vi "My Nonlinear Curve Fit LM bounds.vi"(0 "Y":dbl[](array[numeric]), 1 "f(x,a)":T5, 2 "data":variant, 5 "X":dbl[](array[numeric]), 7 "Weight":dbl[](array[numeric]), 9 "initial parameters":dbl[](array[numeric]), 11 "error in (no error)":errorcluster, 12 "Termination Criteria":T6={"Max Iterations"=1000, "Max Function Calls"=10000, "Max Time"=1000.0, "Function Tolerance"=1e-06, "Parameter Tolerance"=1e-06, "Gradient Tolerance"=1e-06, "Min Lambda"=1e-06, "Max Lambda"=1000000.0, "Initial Tick Count"=0}, 13 "parameter bounds":T3, 14 "method":T4 items=["Least Square", "Least Absolute Residual", "Bisquare"]) -> (3 "Fit Aborted?":bool, 4 "best nonlinear fit":dbl[](array[numeric]), 6 "best fit parameters":dbl[](array[numeric]), 8 "covariance":T7, 10 "Fit Statistics":T1, 15 "error out":errorcluster)   [LabVIEW 2019]
uses:
  <vilib>/Analysis/Matrix/Datatypes/RealMatrix.ctl
  My Fit Stopping Criteria.ctl
  <vilib>/gmath/NumericalOptimization/LM model function reference.ctl
  <vilib>/Analysis/6fits.llb/Curve Fitting Criteria.ctl
  Fit Statistics.ctl
  Convergence Criteria.ctl
  <vilib>/gmath/NumericalOptimization/LM model function.ctl
  <vilib>/gmath/NumericalOptimization/LM_output select.ctl
  Abort Fit Global.vi
  <vilib>/gmath/NI_Gmath.lvlib
  <vilib>/Analysis/NI_AALBase.lvlib
  <vilib>/Analysis/Matrix/NI_Matrix.lvlib
  <vilib>/Analysis/NI_AALPro.lvlib
panel:
  out "Lambda Chart":dbl(graph)
  out "Parameters Gradient Chart":dbl[][](graph)
  in  "Repeat Fit N times (2)":i32=2
  in  "Reset Charts":bool
  out "Chi2 Chart":dbl(graph)
  out "Parameters Graph":dbl[](graph)
  in  "Delay (ms)":i32
  in  "Debug":bool
  out "Parameters Chart":dbl[][](graph)
  out "Function & Fit Graph":cluster{"New Coefficients":dbl[]}[](graph)
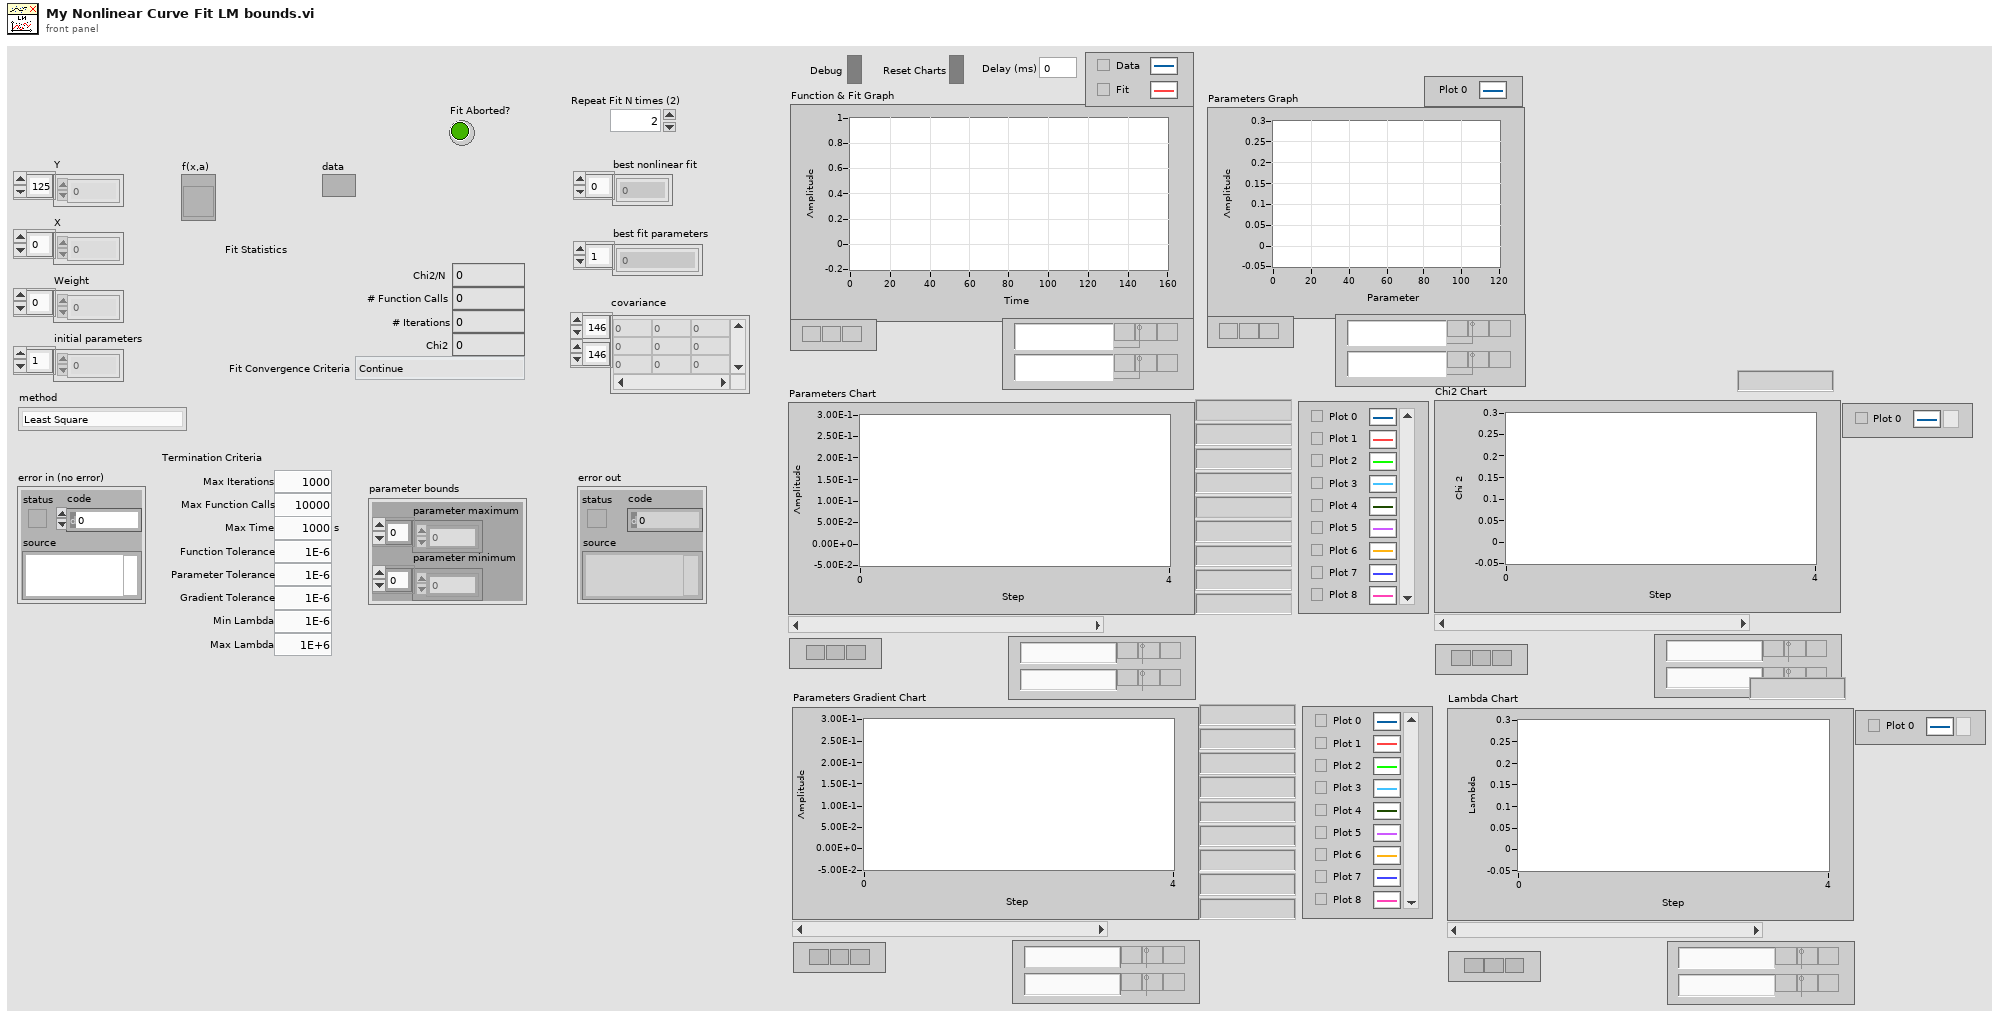
[diagram p1: front panel]
types:
  T1 = typedef "Fit Statistics.ctl" = cluster{"# Iterations":i32, "# Function Calls":i32, "Chi2":dbl, "Chi2/N":dbl, "Fit Convergence Criteria":T2}
  T2 = typedef "Convergence Criteria.ctl" = enum16{"Continue", "Tolerances Exceeded", "Max Time Exceeded", "Max Iterations Exceeded", "Max Function Evaluations Exceeded", "Scale Range Exceeded"}
  T3 = cluster{"parameter minimum":dbl[], "parameter maximum":dbl[]}
  T4 = typedef "NI_AALPro.lvlib/Curve Fitting Criteria.ctl" = u16
  T5 = typedef "NI_Gmath.lvlib/LM model function reference.ctl" = refnum<vi>
  T6 = typedef "My Fit Stopping Criteria.ctl" = cluster{"Max Iterations":i32, "Max Function Calls":i32, "Max Time":dbl[unit], "Function Tolerance":dbl, "Parameter Tolerance":dbl, "Gradient Tolerance":dbl, "Min Lambda":dbl, "Max Lambda":dbl, "Initial Tick Count":u32}
  T7 = typedef "NI_Matrix.lvlib/RealMatrix.ctl" = dbl[][]
  T8 = typedef "NI_Gmath.lvlib/LM model function.ctl" = cluster{"f(x,a)":T5, "data":variant}
  T9 = typedef "NI_Gmath.lvlib/LM_output select.ctl" = cluster{"model function":bool, "gradient":bool}
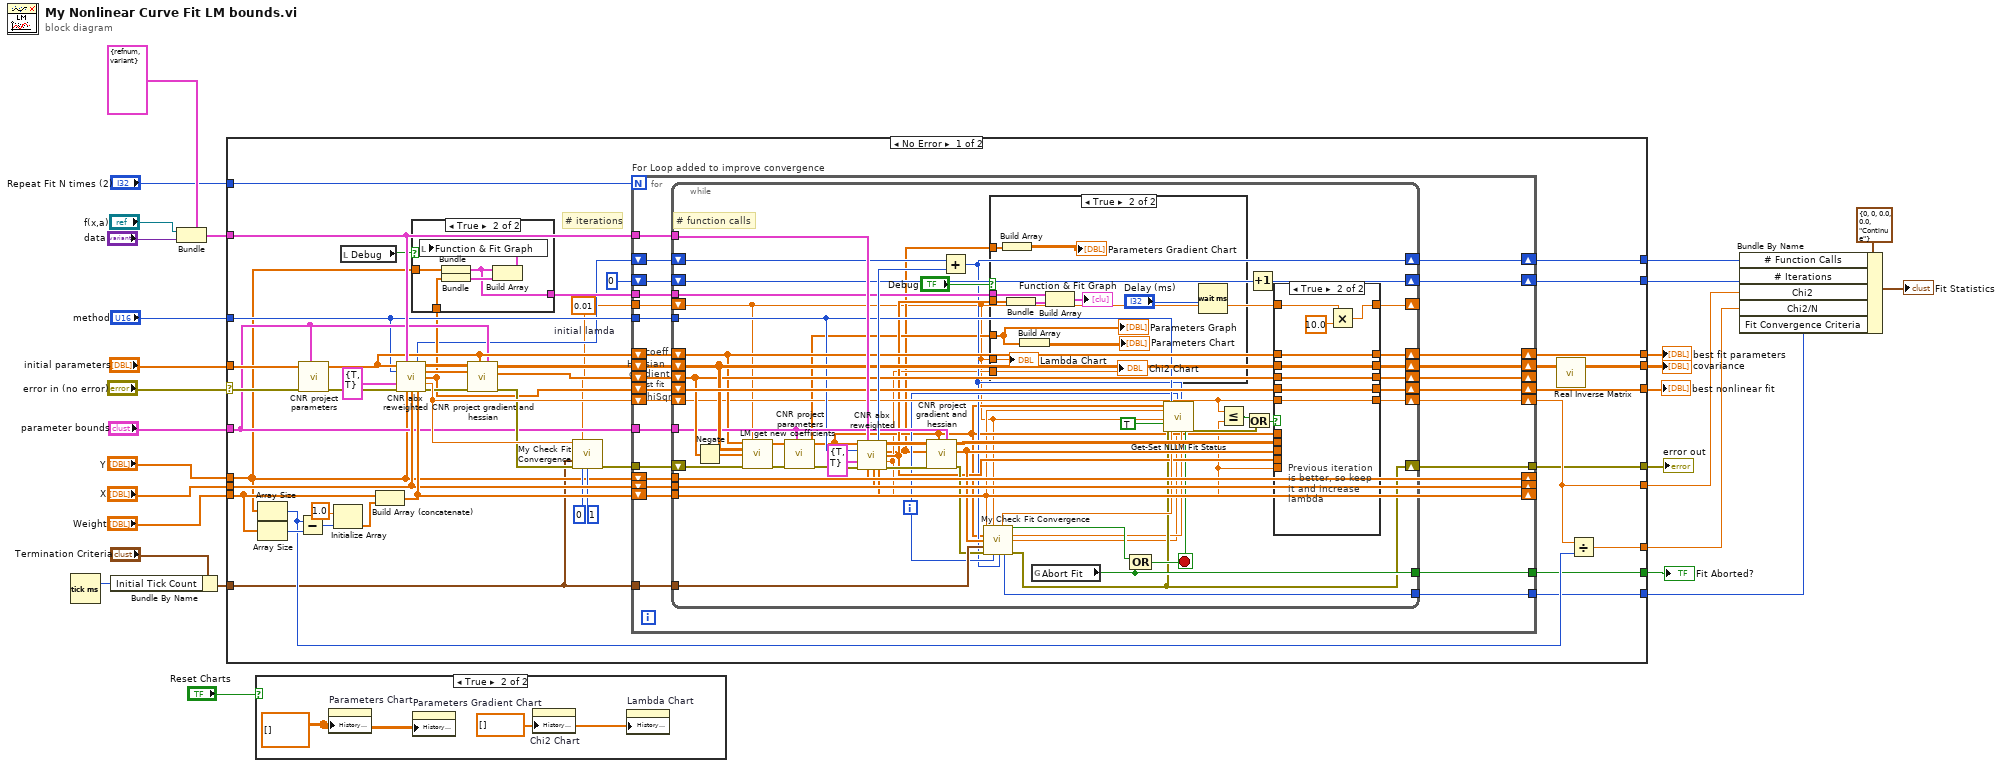
[diagram p0: block diagram]
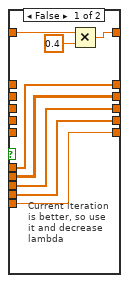
[diagram p4: hidden frame]
diagram:
  n1 = Tick Count (ms)() -> (millisecond timer value=w6:u32)
  n2 = Bundle By Name(cluster="Termination Criteria", "Initial Tick Count"=w6) -> (w5:T6)
  n3 = Bundle(cluster=T8 {"f(x,a)"=refnum, "data"=variant} ("model function"), "f(x,a)"="f(x,a)", "data"="data") -> (w17:T8)
  n4 = case shown="No Error" "error in (no error)" {
    selector: "error in (no error)" -> [w52 w188]
    tunnel: [w55 _] -> w28
    tunnel: [w73 _] -> w8
    tunnel: "initial parameters" -> [w53 _]
    tunnel: [w62 _] -> w26
    tunnel: [w71 _] -> w25
    tunnel: "Weight" -> [w67 _]
    tunnel: "Y" -> [w40 _]
    tunnel: w5 -> [w33 _]
    tunnel: "X" -> [w63 _]
    tunnel: [w32 w188] -> w21
    tunnel: w17 -> [w64 _]
    tunnel: [w57 _] -> w12
    tunnel: "method" -> [w42 _]
    tunnel: "parameter bounds" -> [w45 _]
    tunnel: [w41 _] -> w13
    tunnel: [w36 _] -> w9
    tunnel: [w34 _] -> w10
    tunnel: "Repeat Fit N times (2)" -> [w30 _]
    tunnel: [w29 _] -> w1
    frame No Error {
      w31 = 0.01  # initial lamda
      # "# iterations"
      n5 = Array Size(array=w40) -> (size(s)=w54:i32)
      n6 = Array Size(array=w67) -> (size(s)=w70:i32)
      n7 = Subtract(x=w54, y=w70) -> (x-y=w69:i32)
      n8 = call <vilib>:"CNR project parameters.vi"("bounds"=w45, "error in"=w52, "parameters"=w53) -> ("error out"=w51:errorcluster, "projected parameters"=w46:dbl[])  [unwired: 7 out]
      n9 = Initialize Array(1.0, w69) -> (w68:dbl[])
      n10 = local read "Debug"() -> (w37:bool)
      n11 = Build Array (concatenate)(w67, w68) -> (w74:dbl[])
      n12 = call <vilib>:"CNR abx reweighted.vi"("parameters"=w46, "model function"=w64, "method"=w42, "output control"=T9 {"model function"=TRUE, "gradient"=TRUE}, "error in (no error)"=w51, "Y"=w40, "X"=w63, "Weight"=w74) -> ("number of function calls"=w35:i32, "Hessian"=w48:T7, "gradient"=w47:dbl[], "best fit"=w38:dbl[], "chiSqr"=w66:dbl, "error out"=w50:errorcluster)  [unwired: 1 in, 1 out]
      n13 = case shown="True" w37 {
        tunnel: w40 -> [_ w187]
        tunnel: [_ w184] -> w39
        tunnel: w38 -> [_ w186]
        frame False {
        }
        frame True {
          n14 = Bundle("Y"=w187) -> (w184:cluster{"Y":dbl[]})  [unwired: 1 in]
          n15 = Bundle("best fit"=w186) -> (w185:cluster{"best fit":dbl[]})  [unwired: 1 in]
          n16 = Build Array(w184, w185) -> (w183:cluster{"best fit":dbl[]}[])
          n17 = local write "Function & Fit Graph"(w183) -> ()
        }
      }
      n18 = call <vilib>:"CNR project gradient and hessian.vi"("bounds"=w45, "projected parameters"=w46, "error in"=w50, "gradient"=w47, "Hessian"=w48) -> ("error out"=w49:errorcluster, "projected gradient"=w43:dbl[], "projected Hessian"=w44:T7)  [unwired: 1 in, 3 out]
      n19 = call "My Check Fit Convergence.vi"("Chi 2"=w66, "Lambda"=w31, "my stopping criteria"=w33, "Error In"=w49, "current iteration"=0, "number of function evaluations"=1) -> ("error out"=w65:errorcluster)  [unwired: 4 in, 5 out]
      n20 = for "For Loop added to improve convergence" {
        N: w30 -> [_]
        tunnel: w64 -> [w99]
        tunnel: w45 -> [w92]
        tunnel: w42 -> [w89]
        tunnel: [w88] -> w41
        tunnel: w39 -> [w87]
        tunnel: w33 -> [w82]
        shift-right: [w85] -> w36
        shift-left: w66 -> [w101]
        shift-right: [w95] -> w57
        shift-left: w35 -> [w84]
        shift-right: [w83] -> w34
        shift-left: 0 -> [w96]
        tunnel: w31 -> [w81]
        shift-right: [w94] -> w55
        shift-left: w46 -> [w93]
        shift-right: [w97] -> w59
        shift-left: w44 -> [w91]
        shift-right: [w80] -> _
        shift-left: w43 -> [w90]
        shift-right: [w98] -> w62
        shift-left: w38 -> [w86]
        shift-right: [w79] -> _
        shift-left: w40 -> [w79]
        shift-right: [w78] -> _
        shift-left: w63 -> [w78]
        shift-right: [w77] -> _
        shift-left: w74 -> [w77]
        tunnel: [w75] -> w29
        tunnel: w65 -> [w100]
        tunnel: [w76] -> w32
        # "# function calls"
        # "best fit"
        # "chiSqr"
        # "gradient"
        # "Hessian"
        # "coeff"
        n21 = while {
          tunnel: w78 -> [w150]
          tunnel: w79 -> [w119]
          tunnel: w77 -> [w149]
          shift-left: w101 -> [w123]
          shift-right: [w137] -> w85
          shift-left: w90 -> [w143]
          shift-right: [w153] -> w80
          shift-left: w91 -> [w144]
          shift-right: [w154] -> w97
          shift-left: w93 -> [w125]
          shift-right: [w138] -> w94
          shift-left: w81 -> [w102]
          shift-right: [w151] -> _
          shift-right: [w110] -> w76
          shift-left: w100 -> [w152]
          tunnel: w99 -> [w148]
          tunnel: w82 -> [w140]
          shift-right: [w112] -> w95
          shift-left: w84 -> [w147]
          shift-right: [w145] -> w98
          shift-left: w86 -> [w146]
          shift-right: [w114] -> w83
          shift-left: w96 -> [w115]
          tunnel: w89 -> [w124]
          tunnel: w92 -> [w131]
          tunnel: [w126] -> w88
          tunnel: w87 -> [w118]
          tunnel: [w104] -> w75
          i -> [w113]
          stop <- w111 stop-if-true
          n22 = Negate(x=w143) -> (-x=w127:dbl[])
          n23 = call <vilib>:"LM get new coefficients.vi"("Coefficients"=w125, "lamda"=w102, "Alpha"=w144, "Beta"=w127, "error in (no error)"=w152) -> ("New Coefficients"=w120:dbl[], "error out"=w136:errorcluster)  [unwired: 9 out]
          n24 = call <vilib>:"CNR project parameters.vi"("bounds"=w131, "error in"=w136, "parameters"=w120) -> ("error out"=w135:errorcluster, "projected parameters"=w107:dbl[])  [unwired: 7 out]
          n25 = call <vilib>:"CNR abx reweighted.vi"("parameters"=w107, "model function"=w148, "method"=w124, "output control"=T9 {"model function"=TRUE, "gradient"=TRUE}, "error in (no error)"=w135, "Y"=w119, "X"=w150, "Weight"=w149) -> ("number of function calls"=w155:i32, "Hessian"=w130:T7, "gradient"=w103:dbl[], "best fit"=w116:dbl[], "chiSqr"=w106:dbl, "error out"=w134:errorcluster)  [unwired: 1 in, 1 out]
          n26 = call <vilib>:"CNR project gradient and hessian.vi"("bounds"=w131, "projected parameters"=w107, "error in"=w134, "gradient"=w103, "Hessian"=w130) -> ("error out"=w133:errorcluster, "projected gradient"=w132:dbl[], "projected Hessian"=w129:T7)  [unwired: 1 in, 3 out]
          n27 = Add(x=w147, y=w155) -> (x+y=w112:i32)
          n28 = call "My Check Fit Convergence.vi"("Chi 2"=w106, "Lambda"=w102, "Parameters"=w107, "gradient"=w132, "my stopping criteria"=w140, "Error In"=w133, "current iteration"=w113, "number of function evaluations"=w112) -> ("|Delta Chi 2|/Chi 2"=w121:dbl, "stop?"=w139:bool, "|Delta Chi 2|"=w108:dbl, "Max |Delta a| /|a|"=w105:dbl, "Convergence Criterium Reached"=w104:T2, "error out"=w110:errorcluster)  [unwired: 2 in]
          n29 = case shown="True" "Debug" {
            tunnel: w107 -> [_ w159]
            tunnel: w118 -> [_ w166]
            tunnel: w116 -> [_ w163]
            tunnel: w106 -> [_ w161]
            tunnel: w103 -> [_ w160]
            tunnel: w102 -> [_ w156]
            frame False {
            }
            frame True {
              n30 = Build Array(w160) -> (→"Parameters Gradient Chart":dbl[][])
              n31 = Bundle("best fit"=w163) -> (w165:cluster{"best fit":dbl[]})  [unwired: 1 in]
              n32 = Build Array(w159) -> (→"Parameters Chart":dbl[][])
              n33 = Build Array(w166, w165) -> (→"Function & Fit Graph":cluster{"best fit":dbl[]}[])
              n34 = Wait (ms)(milliseconds to wait="Delay (ms)") -> ()  [unwired: 1 out]
              "Parameters Graph" <- w159
              "Chi2 Chart" <- w161
              "Lambda Chart" <- w156
            }
          }
          n35 = global read "Abort Fit Global.vi" "Abort Fit"() -> (w126:bool)
          n36 = Compound Arithmetic op=OR(w139, w126) -> (w111:bool)
          n37 = call "Get-Set NLLM Fit Status.vi"("Fit Parameters"=w107, "chiSqr"=w106, "Lambda"=w102, "Get(F)/Set"=TRUE, "Error In"=w110, "method"=w124, "|Delta Chi 2|/Chi 2"=w121, "# Iterations"=w113, "Max |Delta a| /|a|"=w105, "# Function Calls"=w112, "|Delta Chi 2|"=w108, "Done"=w111) -> ("Error Out"=w109:errorcluster)  [unwired: 6 in, 1 out]
          n38 = Less Or Equal?(x=w123, y=w106) -> (x <= y?=w142:bool)
          n39 = Or(x=w142, y=w109) -> (x .or. y?=w141:bool)
          n40 = Increment(x=w115) -> (x+1=w114:i32)
          n41 = case shown="True" w141 {
            tunnel: [w173 w182] -> w154
            tunnel: w144 -> [_ w182]
            tunnel: [w172 w181] -> w153
            tunnel: w107 -> [w169 _]
            tunnel: w143 -> [_ w181]
            tunnel: w125 -> [_ w180]
            tunnel: [w169 w180] -> w138
            tunnel: [w174 w178] -> w151
            tunnel: w123 -> [_ w179]
            tunnel: w106 -> [w170 _]
            tunnel: [w170 w179] -> w137
            tunnel: w102 -> [w168 w176]
            tunnel: w129 -> [w173 _]
            tunnel: w132 -> [w172 _]
            tunnel: w146 -> [_ w177]
            tunnel: w116 -> [w171 _]
            tunnel: [w171 w177] -> w145
            frame False {
              # "Current iteration\nis better, so use\nit and decrease \nlambda"
              n42 = Multiply(x=w168, y=0.4) -> (x*y=w174:dbl)
            }
            frame True {
              # "Previous iteration\nis better, so keep\nit and increase \nlambda"
              n43 = Multiply(x=w176, y=10.0) -> (x*y=w178:dbl)
            }
          }
        }
      }
      n44 = call <vilib>:"Real Inverse Matrix.vi"("Input Matrix"=w59) -> ("Inverse Matrix"=w71:T7)  [unwired: 1 in, 1 out]
      n45 = Divide(x=w36, y=w54) -> (x/y=w73:dbl)
    }
    frame Error {
    }
  }
  "best fit parameters" <- w28
  "best nonlinear fit" <- w26
  "error out" <- w21
  "covariance" <- w25
  "Fit Aborted?" <- w13
  n46 = case shown="True" "Reset Charts" {
    frame False {
    }
    frame True {
      w189 = dbl[] [] ("History Data")
      w190 = dbl[][] [] ("History Data")
      n47 = property on="Parameters Chart" class="WFChart (strict)"("History Data"=w190) -> ()  [unwired: 2 in, 2 out]
      n48 = property on="Parameters Gradient Chart" class="WFChart (strict)"("History Data"=w190) -> ()  [unwired: 2 in, 2 out]
      n49 = property on="Chi2 Chart" class="WFChart (strict)"("History Data"=w189) -> ()  [unwired: 2 in, 2 out]
      n50 = property on="Lambda Chart" class="WFChart (strict)"("History Data"=w189) -> ()  [unwired: 2 in, 2 out]
    }
  }
  n51 = Bundle By Name(cluster=T1 {"# Iterations"=0, "# Function Calls"=0, "Chi2"=0.0, "Chi2/N"=0.0, "Fit Convergence Criteria"=enum."Continue"} ("Fit Statistics"), "# Function Calls"=w12, "# Iterations"=w10, "Chi2"=w9, "Chi2/N"=w8, "Fit Convergence Criteria"=w1) -> (→"Fit Statistics":T1)
